vi "sturen_snelheid_regelen.vi"() -> ()   [LabVIEW 2019]
panel:
  out "Snelheid motor rechts":dbl(knob) scale=0.0..10.0
  out "Doet hij dit?":string
  in  "linksafslaan":bool
  out "Doet hij dit?":string
  in  "Licht":bool
  in  "rechtsafslaan":bool
  in  "snelheid regelen motor rechts":dbl(slide) scale=0.0..10.0
  out "Snelheid motor links":dbl(knob) scale=0.0..10.0
  in  "einde van het programma":bool
  in  "Noodstop":bool
  in  "snelheidregelen motor links":dbl(slide) scale=0.0..10.0
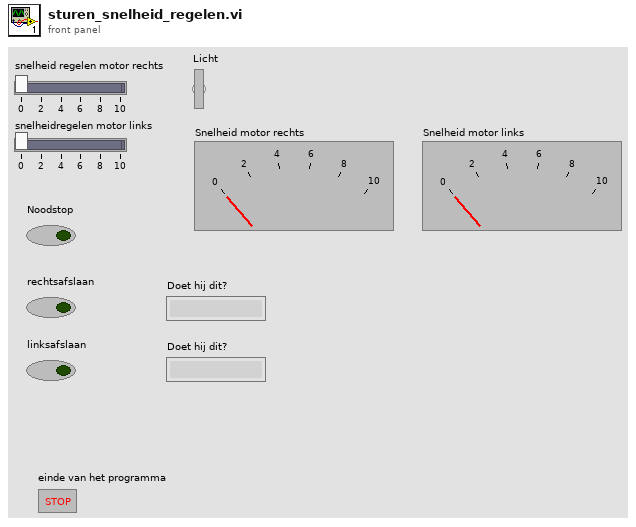
[diagram p1: front panel]
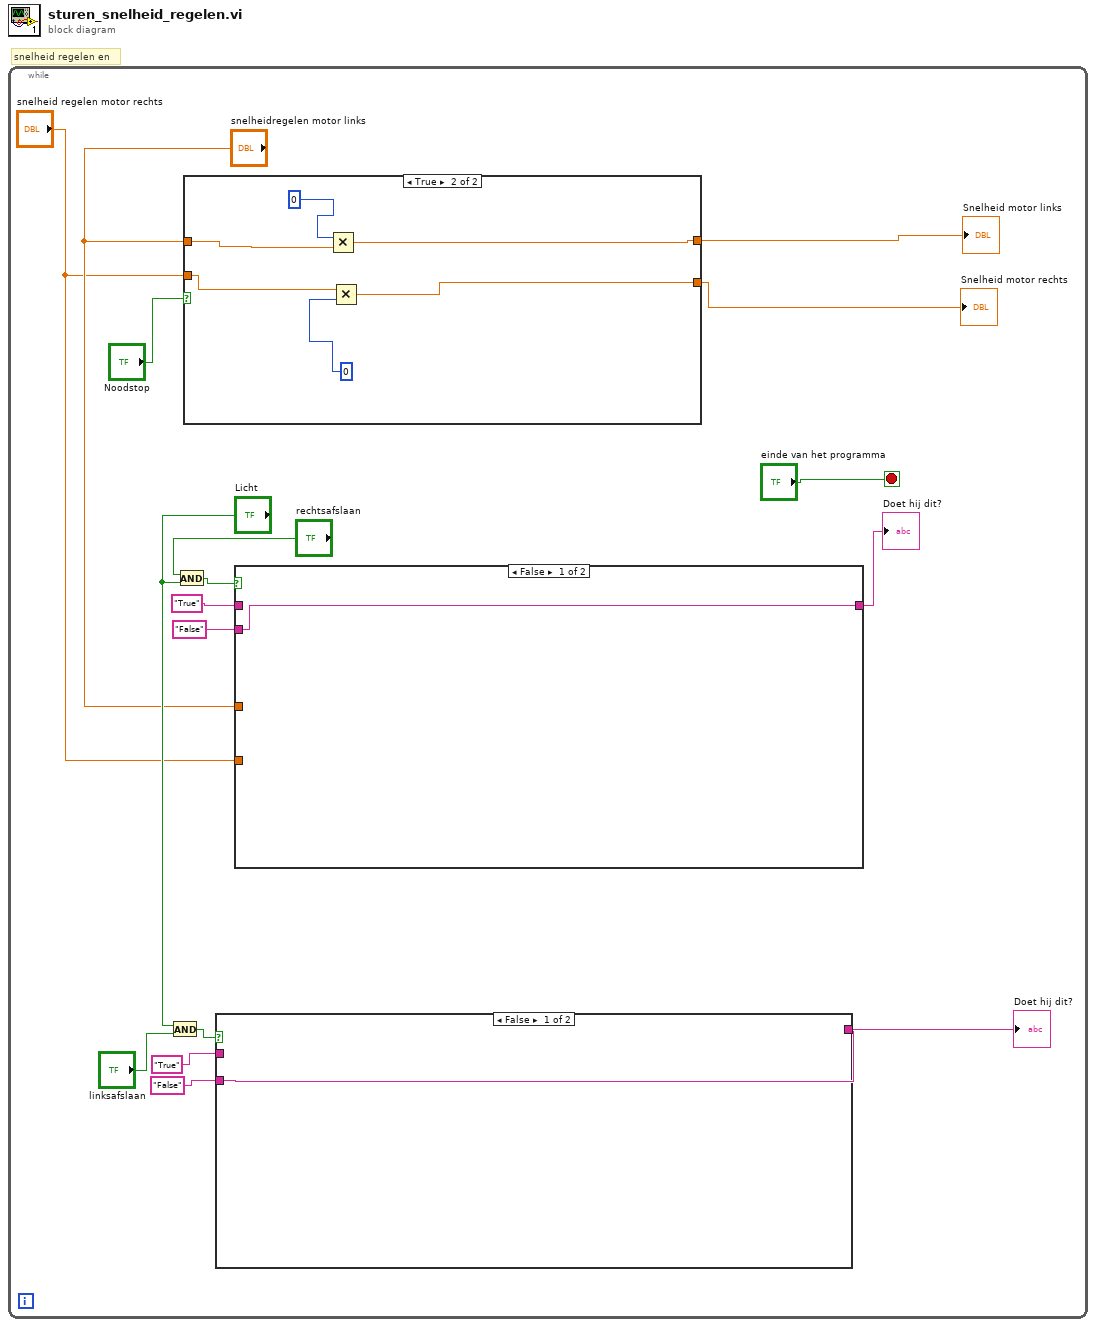
[diagram p0: block diagram]
diagram:
  # "snelheid regelen en"
  n1 = while {
    stop <- "einde van het programma" stop-if-true
    n2 = And(x="Licht", y="linksafslaan") -> (x .and. y?=w6:bool)
    n3 = And(x="rechtsafslaan", y="Licht") -> (x .and. y?=w9:bool)
    n4 = case shown="True" "Noodstop" {
      tunnel: "snelheidregelen motor links" -> [w23 w27]
      tunnel: [w23 w24] -> w16
      tunnel: "snelheid regelen motor rechts" -> [w22 w28]
      tunnel: [w22 w29] -> w7
      frame False {
      }
      frame True {
        n5 = Multiply(x=0, y=w27) -> (x*y=w24:dbl)
        n6 = Multiply(x=w28, y=0) -> (x*y=w29:dbl)
      }
    }
    "Snelheid motor links" <- w16
    "Snelheid motor rechts" <- w7
    n7 = case shown="False" w6 {
      tunnel: "True" -> [_ w19]
      tunnel: [w18 w19] -> w4
      tunnel: "False" -> [w18 _]
      frame False {
      }
      frame True {
      }
    }
    "Doet hij dit?" <- w4
    n8 = case shown="False" w9 {
      tunnel: [w20 w21] -> w14
      tunnel: "False" -> [w20 _]
      tunnel: "True" -> [_ w21]
      tunnel: "snelheid regelen motor rechts" -> [_ _]
      tunnel: "snelheidregelen motor links" -> [_ _]
      frame False {
      }
      frame True {
      }
    }
    "Doet hij dit?" <- w14
  }
